vi "ATM server.vi"   [LabVIEW 2020]
uses:
  <vilib>/Utility/file.llb/Read Delimited Spreadsheet (string).vi
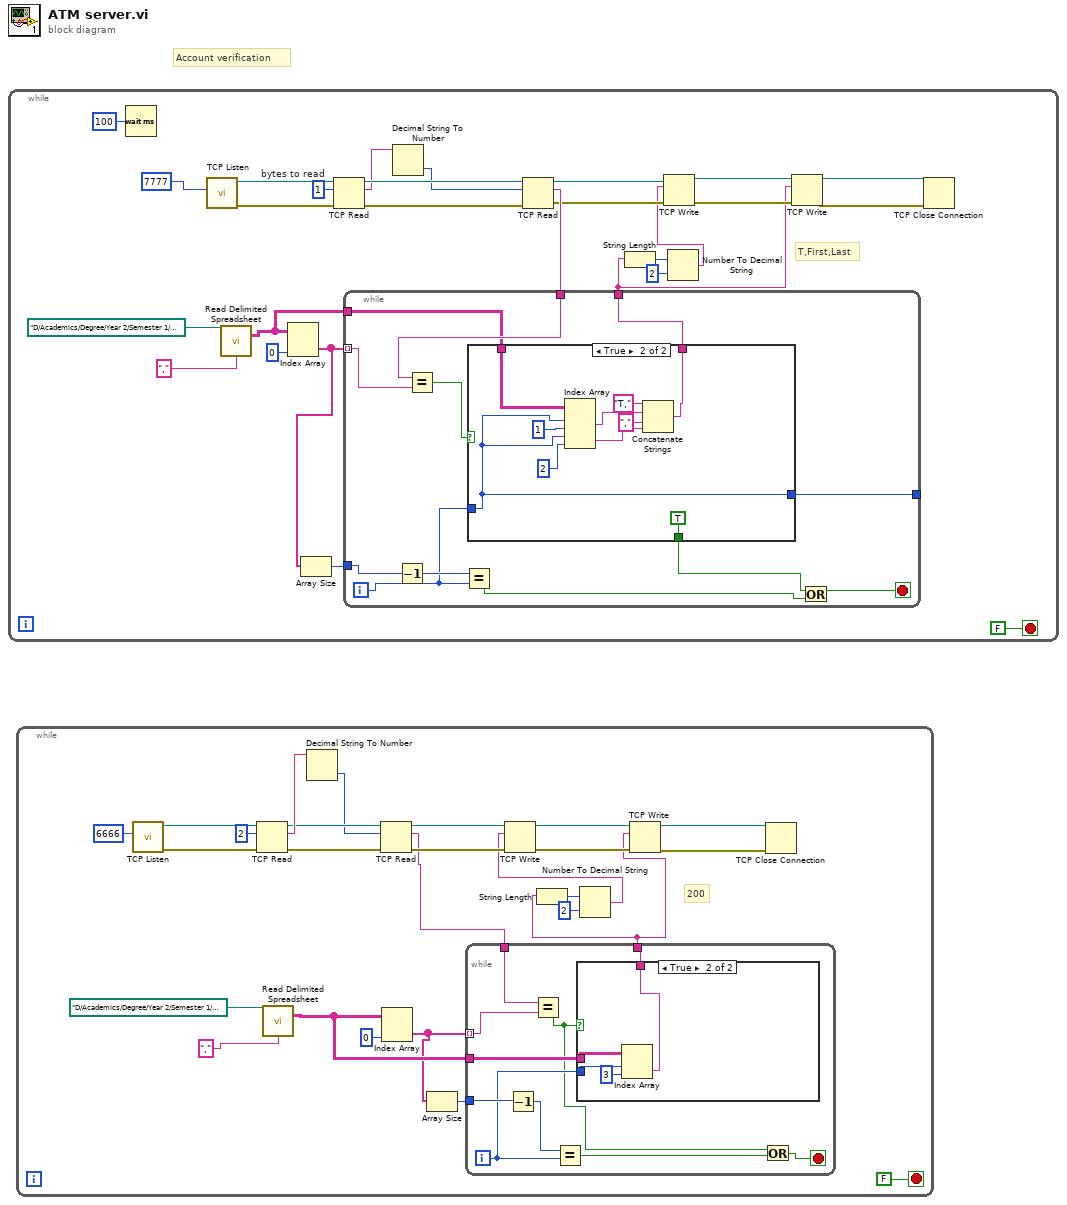
[diagram p0: block diagram]
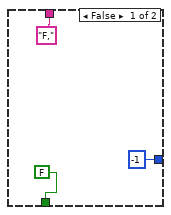
[diagram p3: hidden frame]
diagram:
  # "Account verification"
  n1 = while {
    stop <- FALSE stop-if-true
    w20 = 1  # bytes to read
    # "T,First,Last"
    n2 = Wait (ms)(milliseconds to wait=u32 100) -> ()  [unwired: 1 out]
    n3 = call <vilib>:"TCP Listen.vi"("port"=u16 7777) -> ("error out"=w23:errorcluster, "connection ID"=w25:refnum<k5>)  [unwired: 6 in, 3 out]
    n4 = call-poly <vilib>:"Read Delimited Spreadsheet.vi"("file path (dialog if empty)"=path "D:/Academics/Degree/Year 2/Semester 1/(SPCC) System Programming and Computer Control/Assignment/Accounts.txt", "delimiter (\\t)"="," ("delimiter (\\t)")) -> ("all rows"=w12:string[][])  [unwired: 8 in, 5 out]
    n5 = Index Array(array=w12, index (col)=0 ("disabled index (col)")) -> (element=w14:string[])  [unwired: 1 in]
    n6 = Array Size(array=w14) -> (size(s)=w15:i32)
    n7 = TCP Read(connection ID=w25, bytes to read=w20, error in (no error)=w23) -> (connection ID out=w24:refnum<k5>, data out=w19:string, error out=w22:errorcluster)  [unwired: 2 in]
    n8 = Decimal String To Number(string=w19) -> (number=w18:i32)  [unwired: 2 in, 1 out]
    n9 = TCP Read(connection ID=w24, bytes to read=w18, error in (no error)=w22) -> (connection ID out=w10:refnum<k5>, data out=w11:string, error out=w5:errorcluster)  [unwired: 2 in]
    n10 = while {
      tunnel: w14 -> [w36] mode=indexing
      tunnel: w15 -> [w39]
      tunnel: w12 -> [w31]
      tunnel: w11 -> [w38]
      tunnel: [w29] -> w1
      tunnel: [w28] -> _
      i -> [w30]
      stop <- w34 stop-if-true
      n11 = Decrement(x=w39) -> (x-1=w35:i32)
      n12 = Equal?(x=w38, y=w36) -> (x = y?=w37:bool)
      n13 = Equal?(x=w35, y=w30) -> (x = y?=w33:bool)
      n14 = case shown="True" w37 {
        tunnel: [FALSE TRUE] -> w32
        tunnel: w31 -> [_ w49]
        tunnel: w30 -> [_ w43]
        tunnel: ["F," w46] -> w29
        tunnel: [-1 w43] -> w28
        frame False {
        }
        frame True {
          n15 = Index Array(array=w49, index (row) #1=w43, index (col) #1=1 ("disabled index (col)"), index (row) #2=w43, index (col) #2=2 ("disabled index (col)")) -> (element #1=w48:string, element #2=w47:string)
          n16 = Concatenate Strings("T," ("string"), w48, "," ("string"), w47) -> (w46:string)
        }
      }
      n17 = Or(x=w32, y=w33) -> (x .or. y?=w34:bool)
    }
    n18 = String Length(string=w1) -> (length=w4:i32)
    n19 = Number To Decimal String(number=w4, width (-)=i16 2) -> (decimal integer string=w2:string)
    n20 = TCP Write(connection ID=w10, data in=w2, error in (no error)=w5) -> (connection ID out=w9:refnum<k5>, error out=w6:errorcluster)  [unwired: 1 in, 1 out]
    n21 = TCP Write(connection ID=w9, data in=w1, error in (no error)=w6) -> (connection ID out=w8:refnum<k5>, error out=w7:errorcluster)  [unwired: 1 in, 1 out]
    n22 = TCP Close Connection(connection ID=w8, error in (no error)=w7) -> ()  [unwired: 1 in, 2 out]
  }
  n23 = while {
    stop <- FALSE stop-if-true
    # "200"
    n24 = call <vilib>:"TCP Listen.vi"("port"=u16 6666) -> ("error out"=w68:errorcluster, "connection ID"=w75:refnum<k5>)  [unwired: 6 in, 3 out]
    n25 = TCP Read(connection ID=w75, bytes to read=2, error in (no error)=w68) -> (connection ID out=w74:refnum<k5>, data out=w76:string, error out=w69:errorcluster)  [unwired: 2 in]
    n26 = call-poly <vilib>:"Read Delimited Spreadsheet.vi"("file path (dialog if empty)"=path "D:/Academics/Degree/Year 2/Semester 1/(SPCC) System Programming and Computer Control/Assignment/Accounts.txt", "delimiter (\\t)"="," ("delimiter (\\t)")) -> ("all rows"=w59:string[][])  [unwired: 8 in, 5 out]
    n27 = Decimal String To Number(string=w76) -> (number=w67:i32)  [unwired: 2 in, 1 out]
    n28 = TCP Read(connection ID=w74, bytes to read=w67, error in (no error)=w69) -> (connection ID out=w73:refnum<k5>, data out=w60:string, error out=w70:errorcluster)  [unwired: 2 in]
    n29 = Index Array(array=w59, index (col)=0 ("disabled index (col)")) -> (element=w54:string[])  [unwired: 1 in]
    n30 = Array Size(array=w54) -> (size(s)=w53:i32)
    n31 = while {
      tunnel: w54 -> [w87] mode=indexing
      tunnel: w60 -> [w88]
      tunnel: w59 -> [w86]
      tunnel: [w85] -> w55
      tunnel: w53 -> [w84]
      i -> [w82]
      stop <- w81 stop-if-true
      n32 = Decrement(x=w84) -> (x-1=w83:i32)
      n33 = Equal?(x=w88, y=w87) -> (x = y?=w80:bool)
      n34 = Equal?(x=w83, y=w82) -> (x = y?=w79:bool)
      n35 = case shown="True" w80 {
        tunnel: w86 -> [_ w92]
        tunnel: w82 -> [_ w91]
        tunnel: [_ w89] -> w85
        frame False {
        }
        frame True {
          n36 = Index Array(array=w92, index (row)=w91, index (col)=3 ("disabled index (col)")) -> (element=w89:string)
        }
      }
      n37 = Or(x=w80, y=w79) -> (x .or. y?=w81:bool)
    }
    n38 = String Length(string=w55) -> (length=w57:i32)
    n39 = Number To Decimal String(number=w57, width (-)=i16 2) -> (decimal integer string=w56:string)
    n40 = TCP Write(connection ID=w73, data in=w56, error in (no error)=w70) -> (connection ID out=w72:refnum<k5>, error out=w71:errorcluster)  [unwired: 1 in, 1 out]
    n41 = TCP Write(connection ID=w72, data in=w55, error in (no error)=w71) -> (connection ID out=w77:refnum<k5>, error out=w78:errorcluster)  [unwired: 1 in, 1 out]
    n42 = TCP Close Connection(connection ID=w77, error in (no error)=w78) -> ()  [unwired: 1 in, 2 out]
  }
